vi "CreateError.vi"(5 "Warning":bool, 8 "user error in":errorcluster, 10 "error message (\"\")":string=" is an unallowed value", 11 "command":string=" is an unallowed value") -> (0 "user error  out":errorcluster)   [LabVIEW 2011]
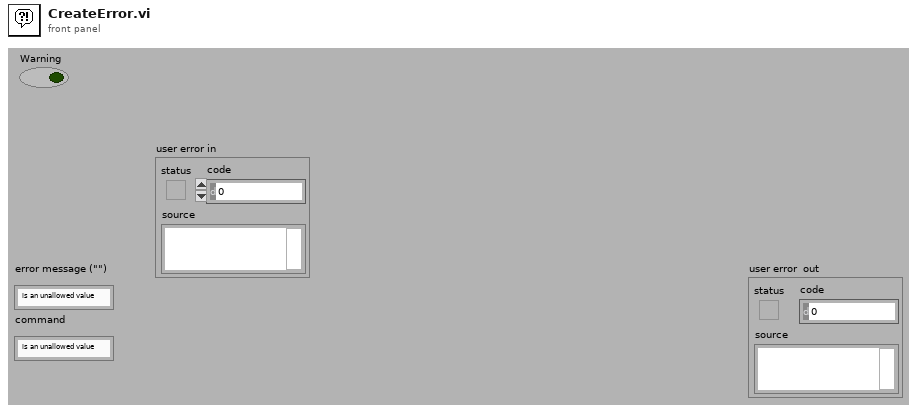
[diagram p1: front panel]
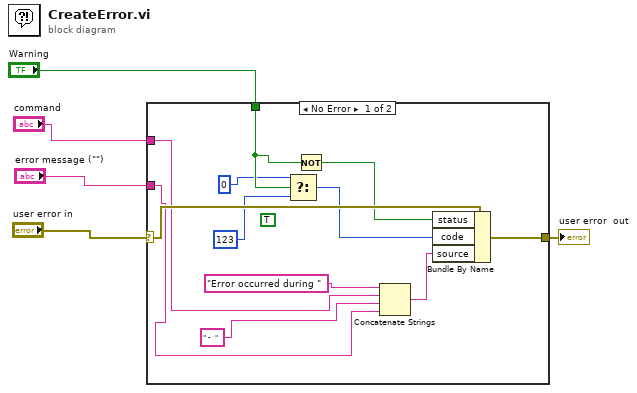
[diagram p0: block diagram]
diagram:
  n1 = case shown="No Error" "user error in" {
    selector: "user error in" -> [w17 w18]
    tunnel: [w11 w18] -> w5
    tunnel: "error message (\"\")" -> [w13 _]
    tunnel: "command" -> [w15 _]
    tunnel: "Warning" -> [w9 _]
    frame No Error {
      (unwired) TRUE ("status")
      n2 = Select(t=0 ("error code (0)"), s=w9, f=123 ("error code (0)")) -> (s? t:f=w6:i32)
      n3 = Not(x=w9) -> (.not. x?=w10:bool)
      n4 = Concatenate Strings("Error occurred during ", w15, " -  ", w13) -> (w12:string)
      n5 = Bundle By Name(cluster=w17, "status"=w10, "code"=w6, "source"=w12) -> (w11:errorcluster)
    }
    frame Error {
    }
  }
  "user error  out" <- w5
